vi "read_write.vi"(5 "Query?":bool, 6 "error in":errorcluster, 8 "Command":string, 9 "VISA handle in":refnum<visa-resource-name>) -> (0 "error out":errorcluster, 2 "Response":string, 3 "VISA handle out":refnum<visa-resource-name>, 4 "TimeoutFlag":bool)   [LabVIEW 2020]
doc: "This VI allows to send a command to the controller SMC 100 and to receive a response via the connection RS232. It is used in each VI."
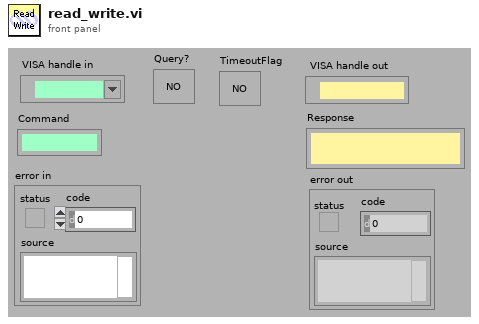
[diagram p1: front panel]
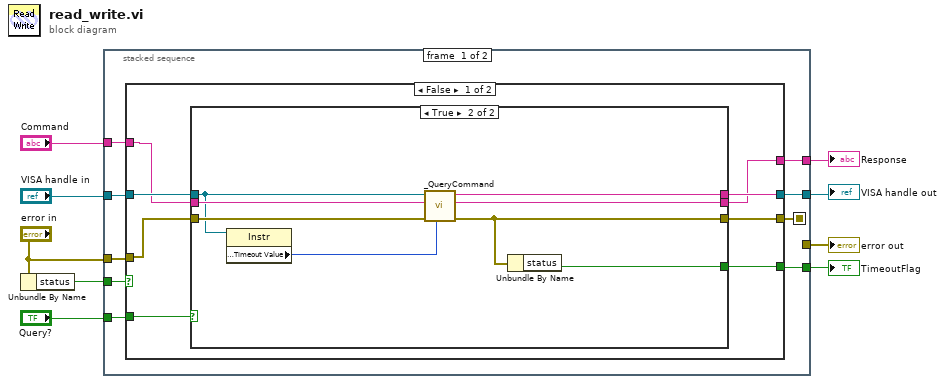
[diagram p0: block diagram]
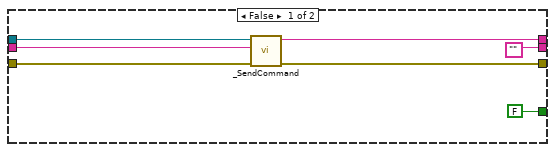
[diagram p2: hidden frame]
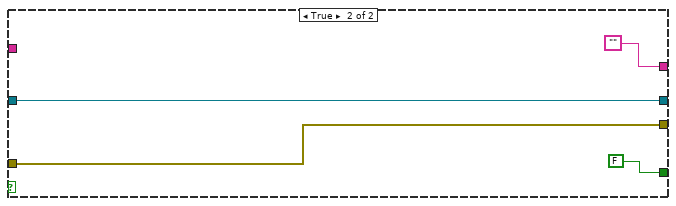
[diagram p3: hidden frame]
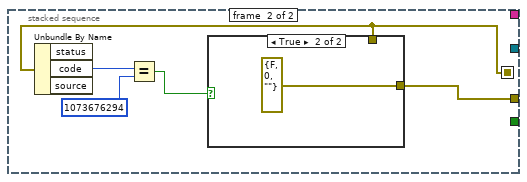
[diagram p4: hidden frame]
diagram:
  n1 = Unbundle By Name("error in") -> ("status"=w8:bool)
  n2 = stacked-sequence {
    seq-local: [w14 _] -> [_ w46]
    tunnel: "VISA handle in" -> [w18 _]
    tunnel: [_ w47] -> w9
    tunnel: w8 -> [w17 _]
    tunnel: "error in" -> [w16 _]
    tunnel: "Query?" -> [w15 _]
    tunnel: "Command" -> [w13 _]
    tunnel: [w12 _] -> w2
    tunnel: [w11 _] -> w4
    tunnel: [w10 _] -> w3
    frame #0 {
      n3 = case shown="False" w17 {
        tunnel: w18 -> [w25 w45]
        tunnel: [w23 w45] -> w12
        tunnel: [w22 w44] -> w14
        tunnel: w16 -> [w24 w44]
        tunnel: [w20 ""] -> w10
        tunnel: [w19 FALSE] -> w11
        tunnel: w15 -> [w26 _]
        tunnel: w13 -> [w21 _]
        frame False {
          n4 = case shown="True" w26 {
            tunnel: w25 -> [w33 w38]
            tunnel: w24 -> [w32 w41]
            tunnel: [w30 w40] -> w23
            tunnel: [w29 w35] -> w22
            tunnel: w21 -> [w31 w39]
            tunnel: ["" w36] -> w20
            tunnel: [FALSE w34] -> w19
            frame False {
              n5 = call "_SendCommand.vi"("error in"=w32, "Command"=w31, "Instrument Channel"=w33) -> ("error out"=w29:errorcluster, "Instrument Channel out"=w30:string)  [unwired: 7 in]
            }
            frame True {
              n6 = property class="Instr"(reference=w38) -> ("General Settings:Timeout Value"=w37:u32)  [unwired: 2 in, 1 out]
              n7 = call "_QueryCommand.vi"("Timeout (ms.) (3000)"=w37, "error in"=w41, "Command"=w39, "Instrument Channel in"=w38) -> ("error out"=w35:errorcluster, "Response"=w36:string, "Instrument Channel out"=w40:string)  [unwired: 5 in]
              n8 = Unbundle By Name(w35) -> ("status"=w34:bool)
            }
          }
        }
        frame True {
        }
      }
    }
    frame #1 {
      n9 = Unbundle By Name(w46) -> ("code"=w50:i32)  [unwired: 2 out]
      n10 = Equal?(x=w50, y=1073676294) -> (x = y?=w49:bool)
      n11 = case shown="True" w49 {
        tunnel: w46 -> [w51 _]
        tunnel: [w51 errorcluster {"status"=FALSE, "code"=0, "source"=""} ("sortie d'erreur 2")] -> w47
        frame False {
        }
        frame True {
        }
      }
    }
  }
  "VISA handle out" <- w2
  "error out" <- w9
  "Response" <- w3
  "TimeoutFlag" <- w4
